vi "Main.vi"() -> ()   [LabVIEW 2024]
doc: "Use this template to build a simple state machine design pattern. Each state executes code and determines which state to transition to."
uses:
  controls/State.ctl
  controls/Data.ctl
  controls/Config_Settings.ctl
panel:
  in  "Copy Graph Data":bool
  in  "Copy Graph":bool
  in  "Configure (Hardware)":bool
  in  "Save File":bool
  in  "Load File":bool
  out "Data":dbl[](graph)
  in  "Clear Graph":bool
  in  "Reset Config Settings":bool
  in  "Analyze Data":bool
  in  "Acquire Data":bool
  in  "Configure (Simulated)":bool
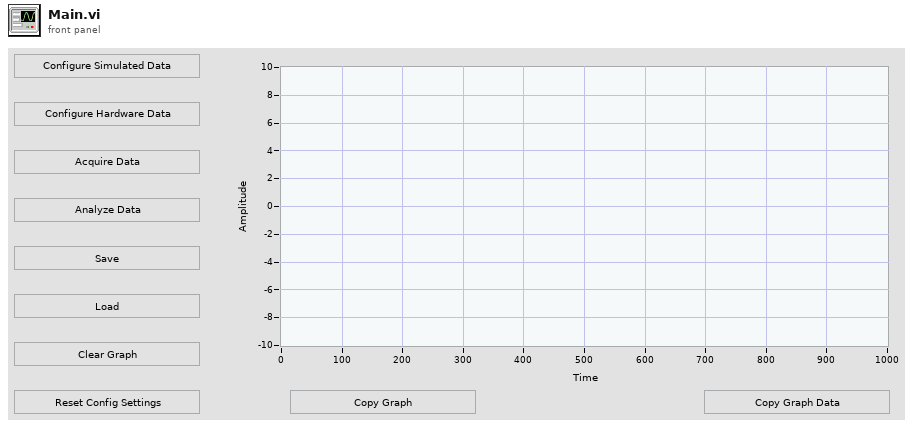
[diagram p1: front panel]
types:
  T1 = typedef "Data.ctl" = cluster{"Config Settings":T2, "Data":dbl[]}
  T2 = typedef "Config_Settings.ctl" = cluster{"signal type":enum16{"Sine Wave", "Triangle Wave", "Square Wave", "Sawtooth Wave"}, "Amplitude":dbl, "Frequency":dbl, "Phase":dbl, "Offset":dbl, "Noise Amplitude":dbl, "Square Wave Duty Cycle":dbl, "Sampling Info":cluster{"Samples per Sec":dbl, "Number of Samples":dbl}}
  T3 = typedef "State.ctl" = enum16{"Initialize", "Update Display", "Wait For Event", "Configuration (Simulated)", "Configuration (Hardware)", "Acquire", "Analyze", "Clear Data", "Reset Settings", "Close", "Save", "Load", "Error"}
  T4 = enum16{"Sine Wave", "Triangle Wave", "Square Wave", "Sawtooth Wave"}
  T5 = typedef "file_type.ctl" = enum16{"txt", "csv", "tdms"}
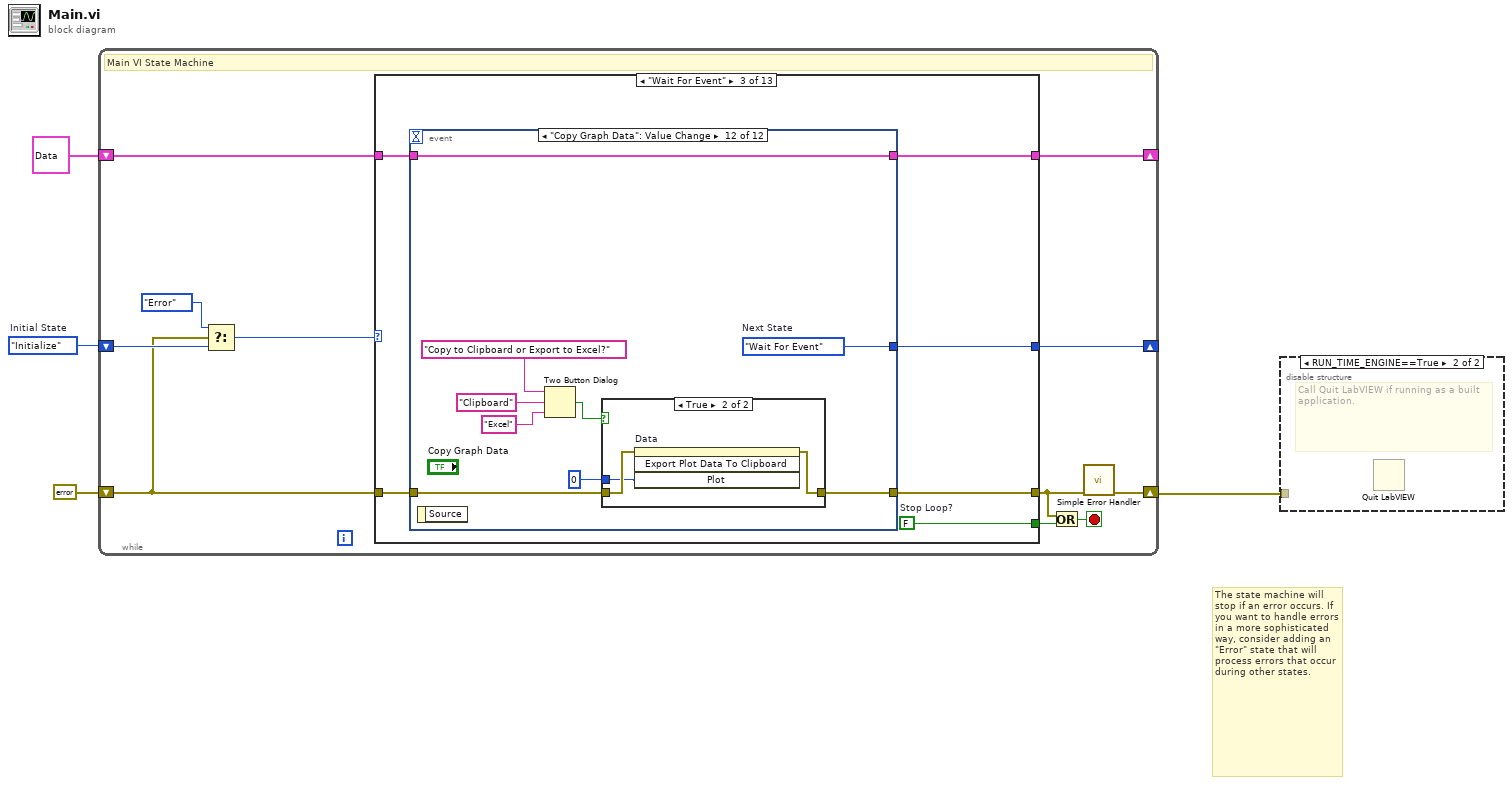
[diagram p0: block diagram]
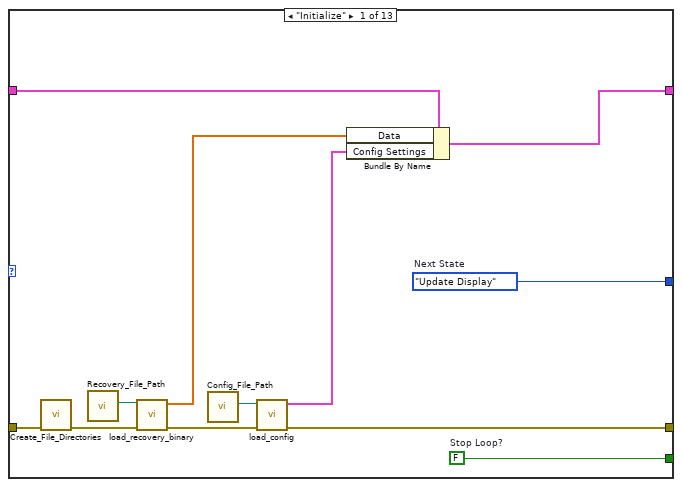
[diagram p3: hidden frame]
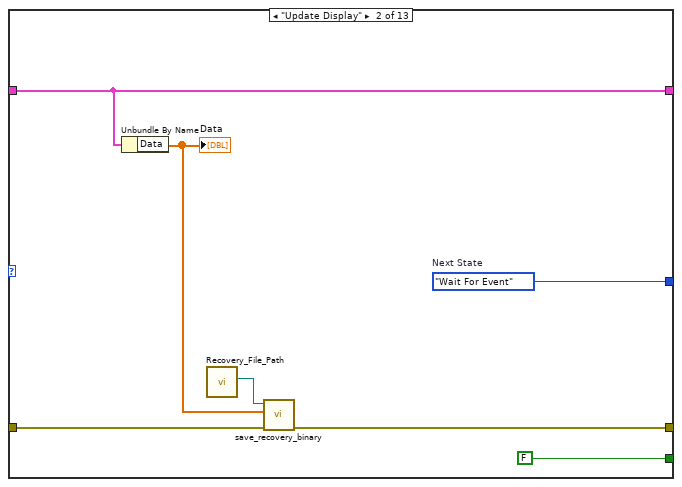
[diagram p4: hidden frame]
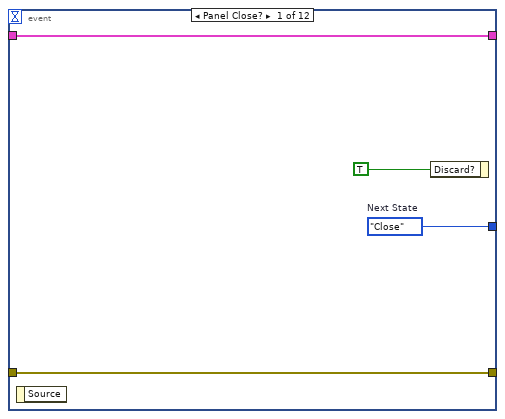
[diagram p5: hidden frame]
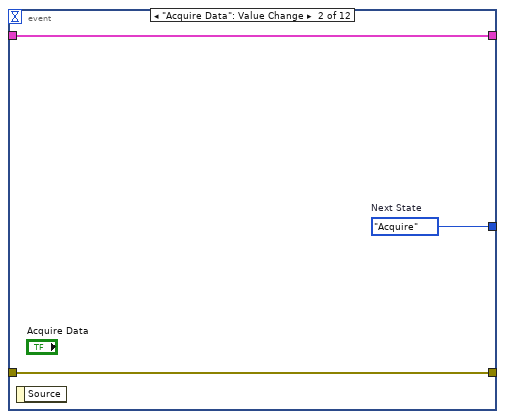
[diagram p6: hidden frame]
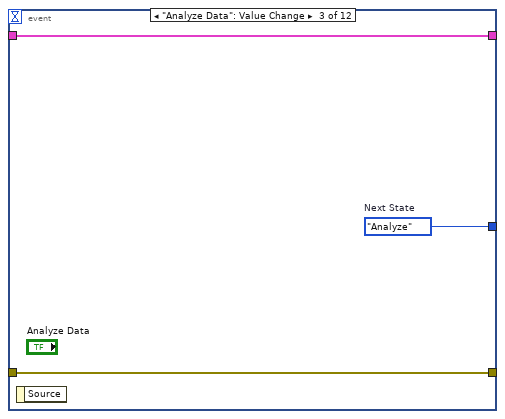
[diagram p7: hidden frame]
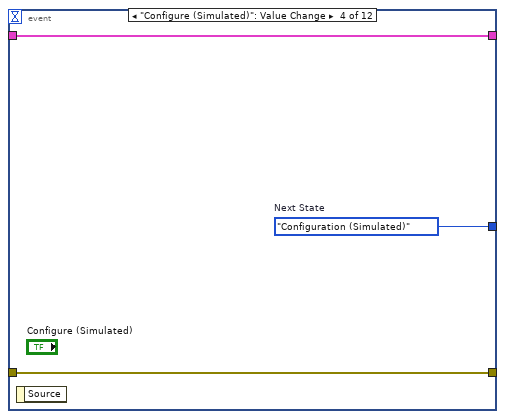
[diagram p8: hidden frame]
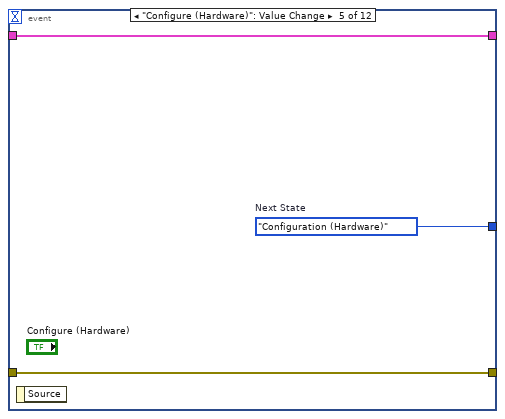
[diagram p9: hidden frame]
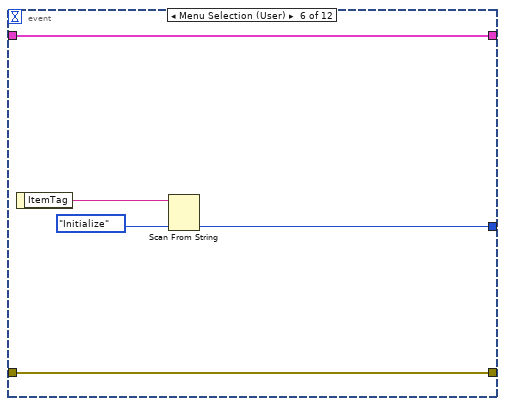
[diagram p10: hidden frame]
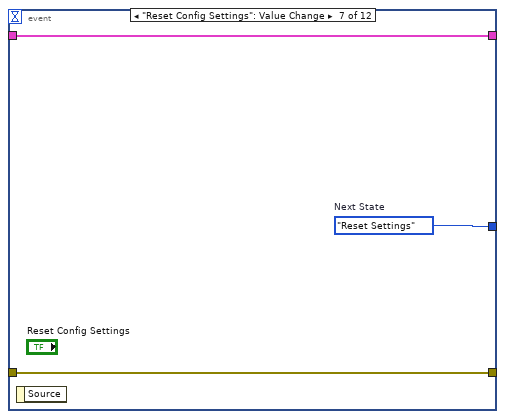
[diagram p11: hidden frame]
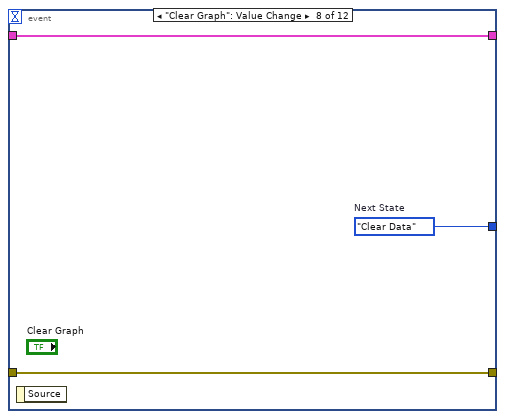
[diagram p12: hidden frame]
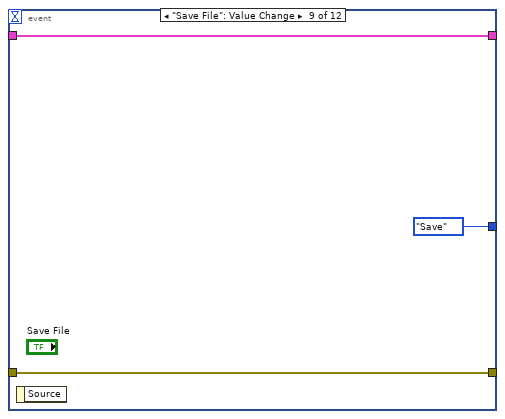
[diagram p13: hidden frame]
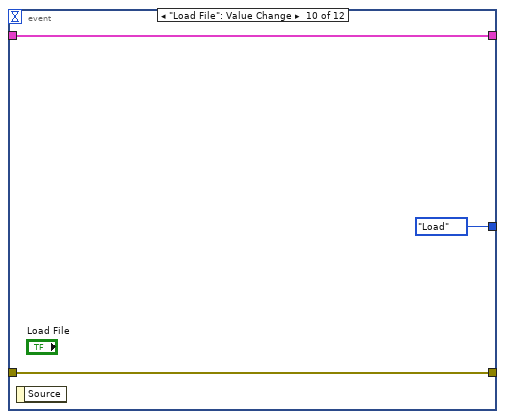
[diagram p14: hidden frame]
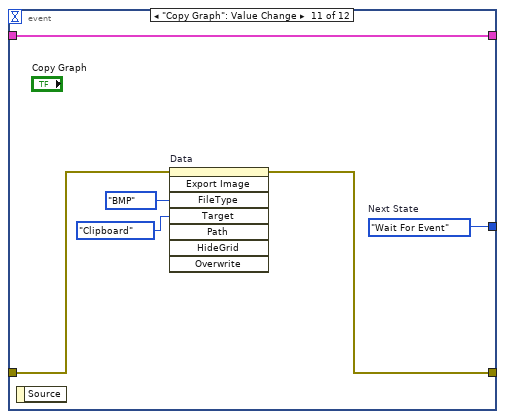
[diagram p15: hidden frame]
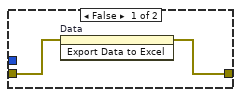
[diagram p16: hidden frame]
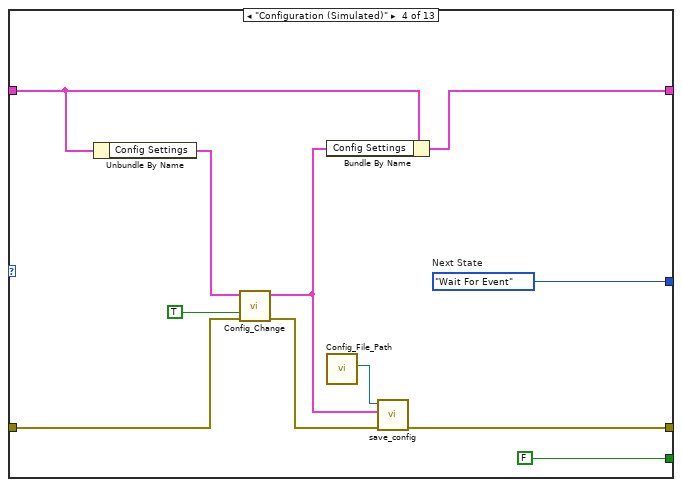
[diagram p17: hidden frame]
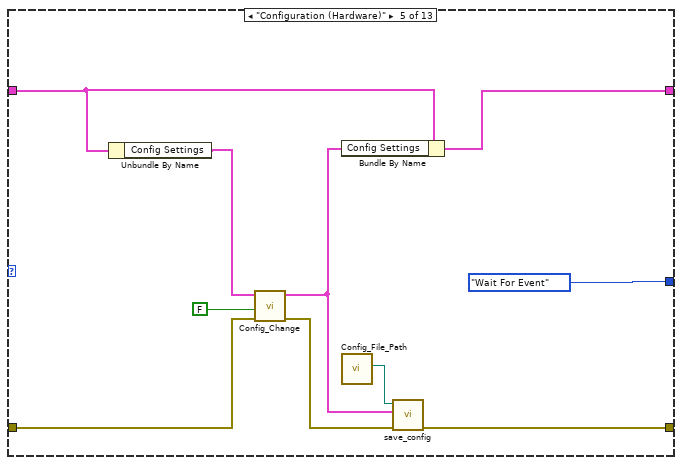
[diagram p18: hidden frame]
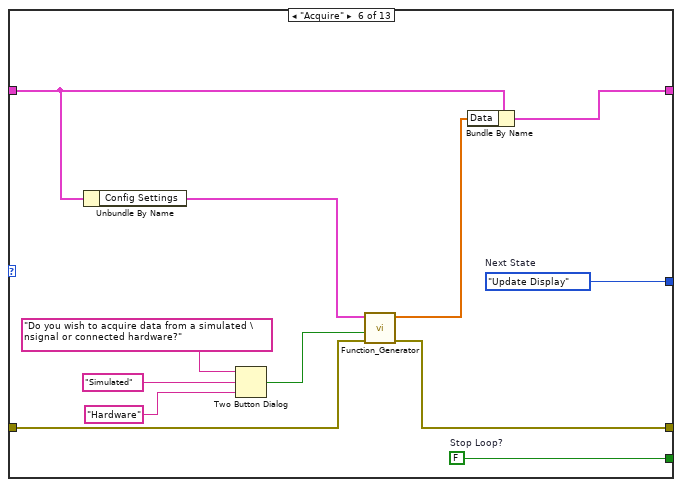
[diagram p19: hidden frame]
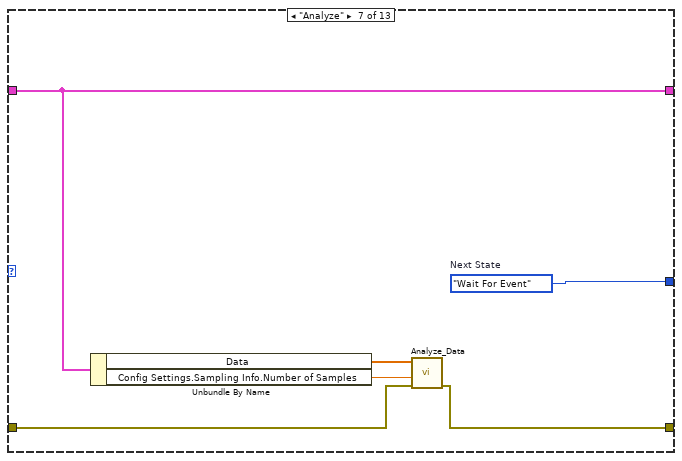
[diagram p20: hidden frame]
diagram:
  w5 = State."Initialize"  # Initial State
  # "The state machine will stop if an error occurs. If you want to handle errors in a more sophisticated way, consider adding an \"Error\" state that will process errors that occur during other states."
  n1 = while {
    shift-right: [w15] -> _
    shift-left: w5 -> [w9]
    shift-right: [w13] -> _
    shift-left: T1 {"Config Settings"={"signal type"=enum."Sine Wave", "Amplitude"=0.0, "Frequency"=0.0, "Phase"=0.0, "Offset"=0.0, "Noise Amplitude"=0.0, "Square Wave Duty Cycle"=0.0, "Sampling Info"={"Samples per Sec"=0.0, "Number of Samples"=0.0}}, "Data"=[]} ("Data") -> [w14]
    shift-right: [w10] -> w2
    shift-left: errorcluster {"status"=FALSE, "code"=0, "source"=""} ("error constant") -> [w8]
    stop <- w11 stop-if-true
    # "Main VI State Machine"
    n2 = Select(t=State."Error", s=w8, f=w9) -> (s? t:f=w6:T3)
    n3 = case shown="\"Wait For Event\"" w6 {
      tunnel: [w27 w34 w40 w104 State."Wait For Event" ("Next State") w126 w132 w135 w149 _ State."Wait For Event" ("Next State") w172 State."Close" ("Next State")] -> w15
      tunnel: [w26 FALSE ("Stop Loop?") w39 FALSE ("Stop Loop?") _ w125 _ _ _ TRUE _ _ _] -> w12
      tunnel: w14 -> [w24 w31 w38 w99 w107 w121 w131 w137 w148 w153 w161 w163 w215]
      tunnel: [w23 w31 w37 w98 w106 w120 w131 w134 w138 w153 w161 w162 w215] -> w13
      tunnel: w8 -> [w25 w32 w36 w101 w110 w123 w129 w136 w150 w152 w154 w168 w214]
      tunnel: [w22 w30 w35 w97 w109 w122 w128 w136 w150 w152 w160 w164 errorcluster {"status"=FALSE, "code"=0, "source"=""} ("error constant")] -> w10
      frame "Initialize" {
        w26 = FALSE  # Stop Loop?
        w27 = State."Update Display"  # Next State
        # "Initialize - Initialize the application."
        n4 = call "Create_File_Directories.vi"("error in (no error)"=w25) -> ("error out"=w19:errorcluster)  [unwired: 10 in]
        n5 = call "Recovery_File_Path.vi"() -> ("Recovery File Path"=w16:path)  [unwired: 11 in]
        n6 = call "load_recovery_binary.vi"("error in (no error)"=w19, "Path"=w16) -> ("error out"=w18:errorcluster, "Data"=w17:dbl[])  [unwired: 8 in]
        n7 = call "Config_File_Path.vi"() -> ("Config File Path"=w20:path)  [unwired: 11 in]
        n8 = call "load_config.vi"("error in (no error)"=w18, "Path"=w20) -> ("error out"=w22:errorcluster, "Config Settings"=w21:T2)  [unwired: 8 in]
        n9 = Bundle By Name(cluster=w24, "Data"=w17, "Config Settings"=w21) -> (w23:T1)
      }
      frame "Update Display" {
        w34 = State."Wait For Event"  # Next State
        n10 = Unbundle By Name(w31) -> ("Data"=w29:dbl[])
        "Data" <- w29
        n11 = call "Recovery_File_Path.vi"() -> ("Recovery File Path"=w28:path)  [unwired: 11 in]
        n12 = call "save_recovery_binary.vi"("error in (no error)"=w32, "Data"=w29, "Path"=w28) -> ("error out"=w30:errorcluster)  [unwired: 8 in]
      }
      frame "Wait For Event" {
        w39 = FALSE  # Stop Loop?
        # "Wait for Event - Use an Event Structure to monitor the user interface for events that run different states of the state machine."
        n13 = event shown="[11] \"Copy Graph Data\": Value Change" {
          selector: _ -> [_ _ _ _ _ _ _ _ _ _ _ _]
          dyn-events: _ -> [_ _ _ _ _ _ _ _ _ _ _ _]
          timeout: _ -> [_ _ _ _ _ _ _ _ _ _ _ _]
          tunnel: [w44 w45 w48 w51 w54 w57 w62 w65 State."Save" ("Next State") State."Load" ("Next State") w76 w84] -> w40
          tunnel: w38 -> [w42 w47 w50 w53 w56 w61 w64 w67 w70 w73 w79 w88]
          tunnel: [w42 w47 w50 w53 w56 w61 w64 w67 w70 w73 w79 w88] -> w37
          tunnel: w36 -> [w43 w46 w49 w52 w55 w60 w63 w66 w69 w72 w78 w82]
          tunnel: [w43 w46 w49 w52 w55 w60 w63 w66 w69 w72 w77 w81] -> w35
          event Panel Close? {
            w44 = State."Close"  # Next State
            n14 = event-data() -> ()  [unwired: 1 in, 1 out]
            n15 = event-data("Discard?"=TRUE) -> ()  [unwired: 1 in, 1 out]
          }
          event "Acquire Data": Value Change {
            w45 = State."Acquire"  # Next State
            n16 = event-data() -> ()  [unwired: 1 in, 1 out]
          }
          event "Analyze Data": Value Change {
            w48 = State."Analyze"  # Next State
            n17 = event-data() -> ()  [unwired: 1 in, 1 out]
          }
          event "Configure (Simulated)": Value Change {
            w51 = State."Configuration (Simulated)"  # Next State
            n18 = event-data() -> ()  [unwired: 1 in, 1 out]
          }
          event "Configure (Hardware)": Value Change {
            w54 = State."Configuration (Hardware)"  # Next State
            n19 = event-data() -> ()  [unwired: 1 in, 1 out]
          }
          event Menu Selection (User) {
            n20 = event-data() -> ("ItemTag"=w59:string)  [unwired: 1 in]
            n21 = Scan From String(input string=w59, default 1=State."Initialize" ("Next State")) -> (output 1=w57:T3)  [unwired: 3 in, 3 out]
          }
          event "Reset Config Settings": Value Change {
            w62 = State."Reset Settings"  # Next State
            n22 = event-data() -> ()  [unwired: 1 in, 1 out]
          }
          event "Clear Graph": Value Change {
            w65 = State."Clear Data"  # Next State
            n23 = event-data() -> ()  [unwired: 1 in, 1 out]
          }
          event "Save File": Value Change {
            n24 = event-data() -> ()  [unwired: 1 in, 1 out]
          }
          event "Load File": Value Change {
            n25 = event-data() -> ()  [unwired: 1 in, 1 out]
          }
          event "Copy Graph": Value Change {
            w76 = State."Wait For Event"  # Next State
            n26 = event-data() -> ()  [unwired: 1 in, 1 out]
            n27 = invoke on="Data" class="WFGraph (strict)" method="Export Image"(error in=w78, "FileType"=enum32{"BMP", "EPS", "EMF", "PICT"}."BMP" ("File Type"), "Target"=enum32{"File", "Clipboard"}."Clipboard") -> (error out=w77:errorcluster)  [unwired: 5 in, 7 out]
          }
          event "Copy Graph Data": Value Change {
            w84 = State."Wait For Event"  # Next State
            n28 = event-data() -> ()  [unwired: 1 in, 1 out]
            n29 = Two Button Dialog(message="Copy to Clipboard or Export to Excel?", 1:"Excel" ("F button name (\"Cancel\")"), 2:"Clipboard" ("T button name (\"OK\")")) -> (T button?=w83:bool)
            n30 = case shown="True" w83 {
              tunnel: w82 -> [w90 w93]
              tunnel: [w89 w92] -> w81
              tunnel: 0 ("Plot") -> [_ w91]
              frame False {
                n31 = invoke on="Data" class="WFGraph (strict)" method="Export Data to Excel"(error in=w90) -> (error out=w89:errorcluster)  [unwired: 2 in, 2 out]
              }
              frame True {
                n32 = invoke on="Data" class="WFGraph (strict)" method="Export Plot Data To Clipboard"(error in=w93, "Plot"=w91) -> (error out=w92:errorcluster)  [unwired: 2 in, 3 out]
              }
            }
          }
        }
      }
      frame "Configuration (Simulated)" {
        w104 = State."Wait For Event"  # Next State
        # "User State 2 - Replace this state with functionality for your own application."
        n33 = Unbundle By Name(w99) -> ("Config Settings"=w102:T2)
        n34 = call "Config_Change.vi"("error in (no error)"=w101, "Simulated Signal ?"=TRUE, "Config In"=w102) -> ("error out"=w100:errorcluster, "Config Out"=w96:T2)  [unwired: 7 in]
        n35 = Bundle By Name(cluster=w99, "Config Settings"=w96) -> (w98:T1)
        n36 = call "Config_File_Path.vi"() -> ("Config File Path"=w95:path)  [unwired: 11 in]
        n37 = call "save_config.vi"("error in (no error)"=w100, "Config Settings"=w96, "Path"=w95) -> ("error out"=w97:errorcluster)  [unwired: 8 in]
      }
      frame "Configuration (Hardware)" {
        n38 = Unbundle By Name(w107) -> ("Config Settings"=w108:T2)
        n39 = call "Config_Change.vi"("error in (no error)"=w110, "Simulated Signal ?"=FALSE, "Config In"=w108) -> ("error out"=w113:errorcluster, "Config Out"=w112:T2)  [unwired: 7 in]
        n40 = Bundle By Name(cluster=w107, "Config Settings"=w112) -> (w106:T1)
        n41 = call "Config_File_Path.vi"() -> ("Config File Path"=w111:path)  [unwired: 11 in]
        n42 = call "save_config.vi"("error in (no error)"=w113, "Config Settings"=w112, "Path"=w111) -> ("error out"=w109:errorcluster)  [unwired: 8 in]
      }
      frame "Acquire" {
        w125 = FALSE  # Stop Loop?
        w126 = State."Update Display"  # Next State
        # "Exit - Exit the application."
        n43 = Unbundle By Name(w121) -> ("Config Settings"=w124:T2)
        n44 = Two Button Dialog(message="Do you wish to acquire data from a simulated \nsignal or connected hardware?", 1:"Hardware" ("F button name (\"Cancel\")"), 2:"Simulated" ("T button name (\"OK\")")) -> (T button?=w115:bool)
        n45 = call "Function_Generator.vi"("error in (no error)"=w123, "Simulated Input?"=w115, "Config Settings"=w124) -> ("error out"=w122:errorcluster, "Data Out"=w119:dbl[])  [unwired: 7 in]
        n46 = Bundle By Name(cluster=w121, "Data"=w119) -> (w120:T1)
      }
      frame "Analyze" {
        w132 = State."Wait For Event"  # Next State
        n47 = Unbundle By Name(w131) -> ("Data"=w130:dbl[], "Config Settings.Sampling Info.Number of Samples"=w127:dbl)
        n48 = call "Analyze_Data.vi"("error in (no error)"=w129, "Number of Samples"=w127, "Data In"=w130) -> ("error out"=w128:errorcluster)  [unwired: 8 in]
      }
      frame "Clear Data" {
        w135 = State."Update Display"  # Next State
        n49 = Bundle By Name(cluster=w137, "Data"=dbl[] []) -> (w134:T1)
      }
      frame "Reset Settings" {
        w149 = State."Wait For Event"  # Next State
        n50 = Bundle By Name(cluster=w148, "Config Settings.signal type"=T4."Sine Wave", "Config Settings.Amplitude"=10.0, "Config Settings.Frequency"=2.0, "Config Settings.Phase"=0.0, "Config Settings.Offset"=0.0, "Config Settings.Noise Amplitude"=0.5, "Config Settings.Square Wave Duty Cycle"=50.0, "Config Settings.Sampling Info.Samples per Sec"=1000.0, "Config Settings.Sampling Info.Number of Samples"=1000.0) -> (w138:T1)
      }
      frame "Close" {
      }
      frame "Save" {
        n51 = Unbundle By Name(w161) -> ("Data"=w158:dbl[])
        n52 = call "Choose_File_Type.vi"("error in (no error)"=w154) -> ("error out"=w155:errorcluster, "OK?"=w156:bool, "File Type Out"=w157:T5)  [unwired: 8 in]
        n53 = call "save_file.vi"("Data"=w158, "error in (no error)"=w155, "Yes/No"=w156, "File Type"=w157) -> ("error out"=w160:errorcluster)  [unwired: 7 in]
      }
      frame "Load" {
        n54 = call "File Dialog"("prompt"="Select a File to Open", "error in"=w168, "pattern (all files)"="*.txt;*.csv;*.tdms" ("pattern label"), "pattern label"="Data Files") -> ("selected path"=w167:path, "cancelled"=w165:bool, "error out"=w166:errorcluster)  [unwired: 8 in, 1 out]
        n55 = case shown="False" w165 {
          tunnel: [w181 State."Wait For Event" ("Next State")] -> w172
          tunnel: w167 -> [w179 _]
          tunnel: w166 -> [w178 w210]
          tunnel: [w174 w209] -> w164
          tunnel: w163 -> [w180 w207]
          tunnel: [w173 w207] -> w162
          frame False {
            n56 = call <vilib>:"Get File Extension.vi"("error in (no error)"=w178, "file"=w179) -> ("error out"=w175:errorcluster, "lowercase file extension"=w177:string, "dup file"=w176:path)  [unwired: 5 in, 2 out]
            n57 = case shown="Default" w177 {
              tunnel: [State."Wait For Event" ("Next State") State."Update Display" ("Next State") State."Update Display" ("Next State") State."Update Display" ("Next State")] -> w181
              tunnel: w180 -> [w182 w188 w195 w202]
              tunnel: w176 -> [_ w191 w198 w205]
              tunnel: w175 -> [w183 w190 w197 w204]
              tunnel: [w183 w189 w196 w203] -> w174
              tunnel: [w182 w186 w193 w201] -> w173
              frame Default {
                n58 = One Button Dialog(message="File type selected is not supported!") -> ()  [unwired: 1 in, 1 out]
              }
              frame "txt" {
                n59 = call "load_txt.vi"("error in (no error)"=w190, "Path"=w191) -> ("error out"=w189:errorcluster, "Data"=w187:dbl[])  [unwired: 8 in]
                n60 = Bundle By Name(cluster=w188, "Data"=w187) -> (w186:T1)
              }
              frame "csv" {
                n61 = call "load_csv.vi"("error in (no error)"=w197, "Path"=w198) -> ("error out"=w196:errorcluster, "Data"=w194:dbl[])  [unwired: 8 in]
                n62 = Bundle By Name(cluster=w195, "Data"=w194) -> (w193:T1)
              }
              frame "tdms" {
                n63 = call "load_tdms.vi"("error in (no error)"=w204, "Path"=w205) -> ("error out"=w203:errorcluster, "Data"=w200:dbl[])  [unwired: 8 in]
                n64 = Bundle By Name(cluster=w202, "Data"=w200) -> (w201:T1)
              }
            }
          }
          frame True {
            n65 = call <vilib>:"Clear Errors.vi"("error in (no error)"=w210, "specific error code to clear (0: all)"=43) -> ("error out"=w209:errorcluster)  [unwired: 4 in, 1 out]
          }
        }
      }
      frame "Error" {
        n66 = call <vilib>:"Simple Error Handler.vi"("error in (no error)"=w214) -> ()  [unwired: 4 in, 5 out]
      }
    }
    n67 = Or(x=w10, y=w12) -> (x .or. y?=w11:bool)
  }
  n68 = call <vilib>:"Simple Error Handler.vi"("error in (no error)"=w2) -> ("error out"=w1:errorcluster)  [unwired: 4 in, 4 out]
  n69 = disable-structure shown="RUN_TIME_ENGINE==True" {
    disable-tunnel: w1 -> [_ _]
    frame condition #0 (active) {
    }
    frame condition #1 {
      # "Call Quit LabVIEW if running as a built application."
      n70 = Quit LabVIEW() -> ()  [unwired: 1 in]
    }
  }
